vi "Next.vi"(8 "Error In":errorcluster, 11 "Reader In":refnum<class "String.lvclass">) -> (0 "Error Out":errorcluster, 1 "End?":bool=TRUE, 2 "Character":u8, 3 "Reader Out":refnum<class "String.lvclass">)   [LabVIEW 2017, in "Mustache.lvlib" / "Readers.lvlib" / "String.lvclass"]
uses:
  String.lvclass
  String.lvclass/String.ctl
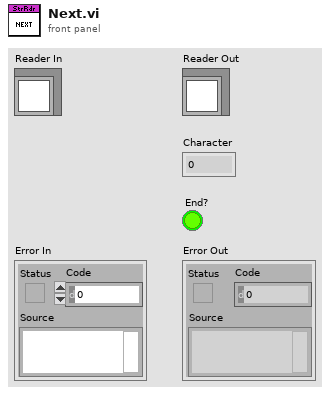
[diagram p1: front panel]
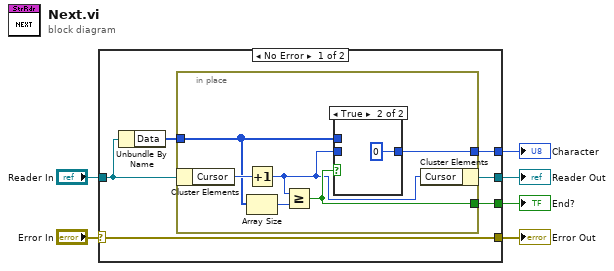
[diagram p0: block diagram]
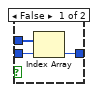
[diagram p2: hidden frame]
diagram:
  n1 = case shown="No Error" "Error In" {
    selector: "Error In" -> [w7 w24]
    tunnel: [w7 w24] -> w5
    tunnel: "Reader In" -> [w11 w23]
    tunnel: [w9 w23] -> w3
    tunnel: [w12 _] -> w2
    tunnel: [w8 _] -> w1
    frame No Error {
      n2 = Unbundle By Name(w11) -> ("Data"=w10:u8[])
      n3 = in-place {
        in-place-border: [w16] -> w12
        in-place-border: w10 -> [w15]
        in-place-border: [w13] -> w8
        n4 = in-place-cluster #1(w11) -> ("Cursor"=w18:i32)
        n5 = Increment(x=w18) -> (x+1=w14:i32)
        n6 = Array Size(array=w15) -> (size(s)=w17:i32)
        n7 = Greater Or Equal?(x=w14, y=w17) -> (x >= y?=w16:bool)
        n8 = case shown="True" w16 {
          tunnel: w15 -> [w21 _]
          tunnel: w14 -> [w20 _]
          tunnel: [w19 u8 0 ("Character")] -> w13
          frame False {
            n9 = Index Array(array=w21, index=w20) -> (element=w19:u8)
          }
          frame True {
          }
        }
        n10 = in-place-cluster #1("Cursor"=w14) -> (w9:refnum<class "String.lvclass">)
      }
    }
    frame Error {
    }
  }
  "Error Out" <- w5
  "Reader Out" <- w3
  "Character" <- w1
  "End?" <- w2
